vi "Arrange AI.vi"(5 "Transformed Calibration Matrix":dbl[][](array[numeric]), 7 "Bias Vector":dbl[](array[numeric])=[-0.07101794332265854, -0.17463348805904388, -0.11016159504652023, 0.02601883001625538, 0.1289764940738678, 0.08259620517492294], 10 "FB data":dbl[](array[numeric]) format="%0.2f", 11 "EDV + Voltage data":dbl[](array[numeric]) format="%0.2f") -> (2 "FIFO Data (7EDV+3Force+4Power+4Voltage)":dbl[](array[numeric]), 3 "UDP Data (7EDV+3Force+4Power)":dbl[](array[numeric]))   [LabVIEW 2021]
uses:
  <vilib>/Analysis/baseanly.llb/A x Vector.vi
  <vilib>/Analysis/NI_AALBase.lvlib
panel:
  out "Raw voltage":dbl[](array[numeric])
  out "Voltages":dbl[](array[numeric])
  out "Forces":dbl[](array[numeric]) format="%.2f"
  out "Endevco":dbl[](array[numeric])
  out "Power":dbl[](array[numeric])
  out "Current":dbl[](array[numeric])
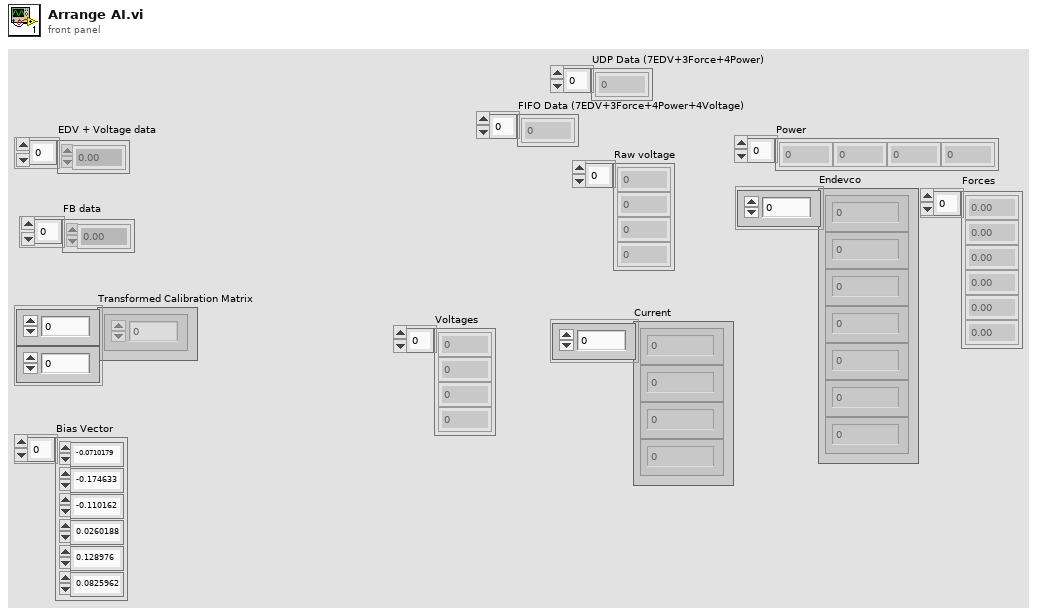
[diagram p1: front panel]
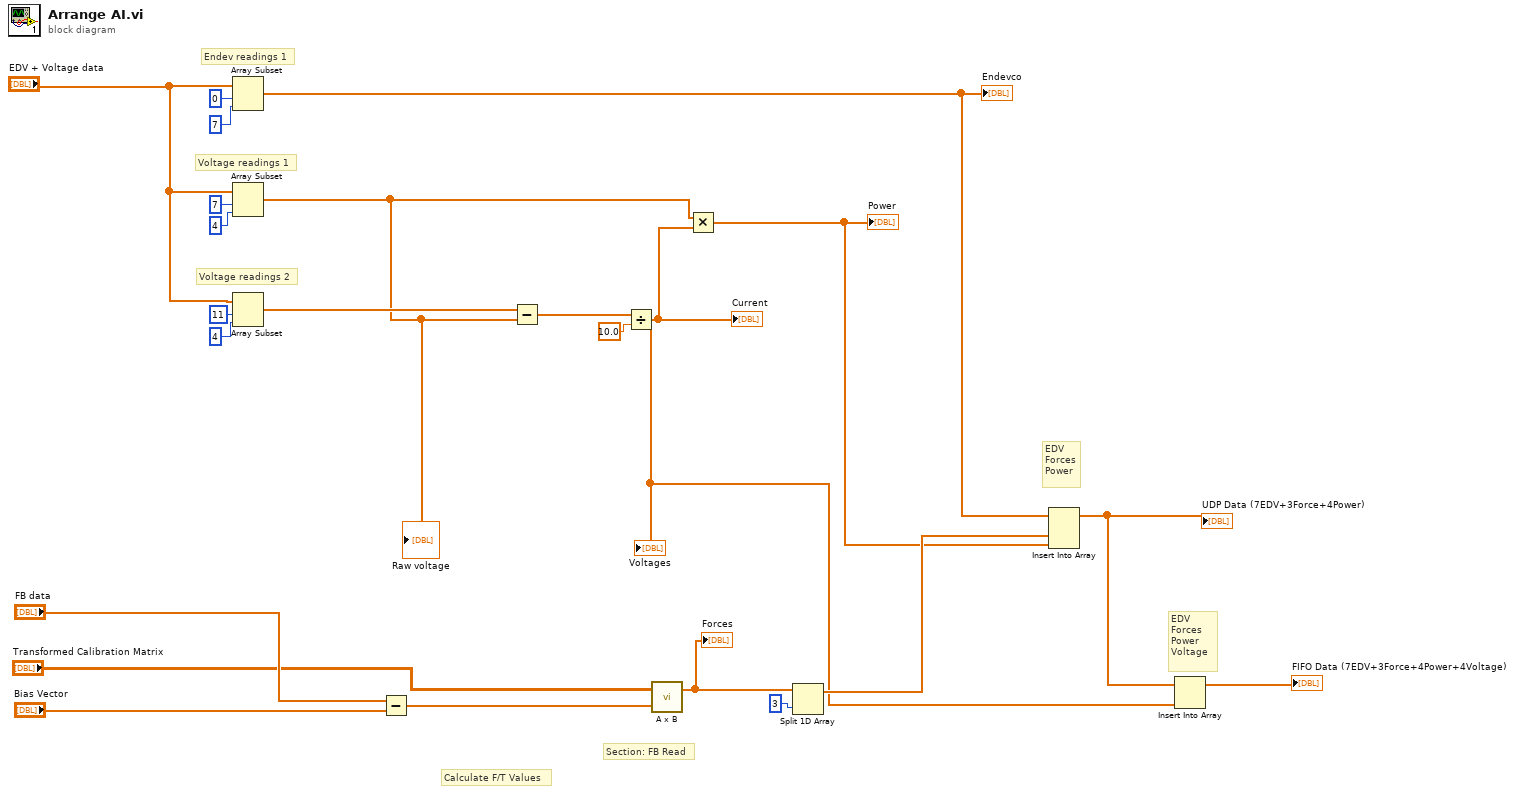
[diagram p0: block diagram]
diagram:
  # "EDV\nForces\nPower\nVoltage"
  # "EDV\nForces\nPower"
  # "Section: FB Read"
  # "Calculate F/T Values"
  # "Endev readings 1"
  # "Voltage readings 2"
  # "Voltage readings 1"
  n1 = Array Subset(array="EDV + Voltage data", index=0, length=7) -> (w4:dbl[])
  "Endevco" <- w4
  n2 = Array Subset(array="EDV + Voltage data", index=7, length=4) -> (w20:dbl[])
  "Raw voltage" <- w20
  n3 = Array Subset(array="EDV + Voltage data", index=11, length=4) -> (w21:dbl[])
  n4 = Subtract(x="FB data", y="Bias Vector") -> (x-y=w12:dbl[])
  n5 = Subtract(x=w21, y=w20) -> (x-y=w2:dbl[])
  "Voltages" <- w2
  n6 = Divide(x=w2, y=10.0) -> (x/y=w19:dbl[])
  "Current" <- w19
  n7 = call-poly <vilib>:"A x B.vi"("Vector"=w12, "A"="Transformed Calibration Matrix") -> ("A x Vector"=w5:dbl[])  [unwired: 1 out]
  "Forces" <- w5
  n8 = Multiply(x=w20, y=w19) -> (x*y=w6:dbl[])
  "Power" <- w6
  n9 = Split 1D Array(array=w5, index=3) -> (first subarray=w7:dbl[])  [unwired: 1 out]
  n10 = Insert Into Array(array=w4, new element #1=w7, new element #2=w6) -> (w3:dbl[])  [unwired: 1 in]
  "UDP Data (7EDV+3Force+4Power)" <- w3
  n11 = Insert Into Array(array=w3, new element=w2) -> (→"FIFO Data (7EDV+3Force+4Power+4Voltage)":dbl[])  [unwired: 1 in]
